vi "Get and Lock Stack.vi"(8 "error in (no error)":errorcluster, 11 "IP Connection in":refnum<class "IP Connection.lvclass">) -> (0 "error out":errorcluster, 2 "Stack":refnum<class "Device.lvclass">[](array[class]), 3 "IP Connection out":refnum<class "IP Connection.lvclass">)   [LabVIEW 2011, in "Tinkerforge.lvlib" / "IP Connection.lvclass"]
doc: "This VI returns the stack and locks the data access."
uses:
  IP Connection.lvclass
  Device/Device.lvclass
  IP Connection.lvclass/IP Connection.ctl
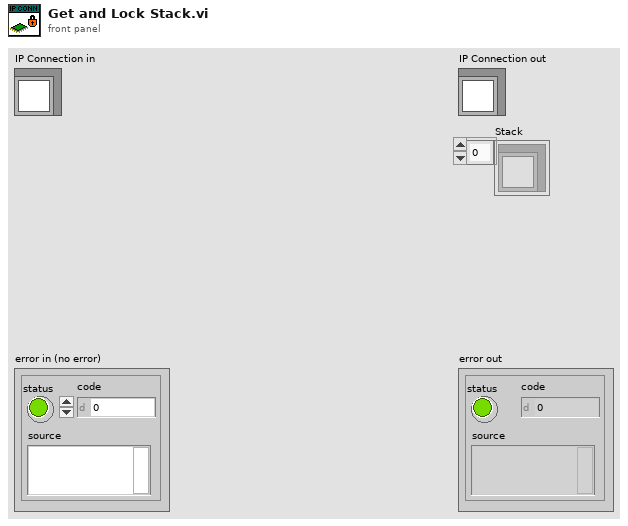
[diagram p1: front panel]
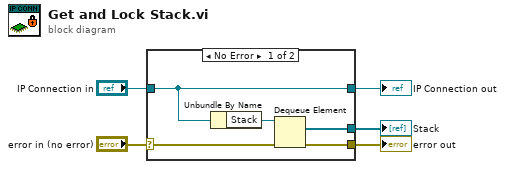
[diagram p0: block diagram]
diagram:
  n1 = case shown="No Error" "error in (no error)" {
    selector: "error in (no error)" -> [w8 w12]
    tunnel: [w7 w12] -> w4
    tunnel: [w10 w11] -> w2
    tunnel: "IP Connection in" -> [w10 w11]
    tunnel: [w6 _] -> w1
    frame No Error {
      n2 = Unbundle By Name(w10) -> ("Stack"=w9:refnum<queue>)
      n3 = Dequeue Element(queue=w9, error in (no error)=w8) -> (element=w6:refnum<class "Device.lvclass">[], error out=w7:errorcluster)  [unwired: 1 in, 2 out]
    }
    frame Error {
    }
  }
  "error out" <- w4
  "IP Connection out" <- w2
  "Stack" <- w1
